vi "UT_002_TOML to LV.vi"() -> ()   [LabVIEW 2020]
uses:
  fb850d28-2e79-48d9-b60b-ba7296d5dbb4.vi
  89a8d650-8cb1-4c84-83d7-77e0f1707b6b.vi
  32d4b0e2-7f7c-42da-9dd6-c3c9d6f0c3e1.vi
  d279671c-9ecb-4521-8644-d889c2403450.vi
  5e8cb647-c85d-4476-b550-d09c056e5780.vi
  c4cfef05-1c91-402b-82a1-7a83dc25bed2.vi
  lib/TOML to LabVIEW.vi
  <vilib>/addons/_JKI Toolkits/Caraya/classes/Assert/Assert True.vi
  <vilib>/addons/_JKI Toolkits/Caraya/classes/Assert/Assert Not Error.vi
  <vilib>/addons/_JKI Toolkits/Caraya/classes/Assert/Assert Error.vi
  <vilib>/addons/_JKI Toolkits/Caraya/classes/Test/Test.lvclass
  <vilib>/addons/_JKI Toolkits/Caraya/classes/Assert/Assert.lvclass
  lib/TOML.lvlib
panel:
  out "error out":errorcluster
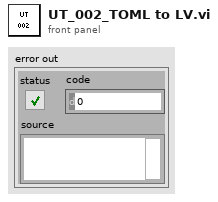
[diagram p1: front panel]
types:
  T1 = cluster{"cluster":cluster{"status":bool, "code":i32, "source":string, "error":errorcluster, "float-array":dbl[], "cluster-array":cluster{"nam":string, "value":dbl}[]}}
  T2 = cluster{"cluster":cluster{"status":bool, "cod":i32, "source":string, "error":errorcluster, "float-array":dbl[], "cluster-array":cluster{"name":string, "value":dbl}[]}}
  T3 = cluster{"status":bool, "code":i32, "source":string, "error":errorcluster, "float-array":dbl[], "cluster-array":cluster{"name":string, "value":dbl}[]}
  T4 = cluster{"cluster":cluster{"status":bool, "code":i32, "source":string, "error":errorcluster, "float-array":dbl[], "cluster-array":cluster{"name":string, "value":dbl}[]}}
  T5 = typedef "TOML.lvlib/TOML Value.ctl" = cluster{"type":enum16{"Table", "Array", "String", "Integer", "Float", "Boolean", "Offset Date-Time", "Local Date-Time", "Local Date", "Local Time", "Path"}, "value":variant}
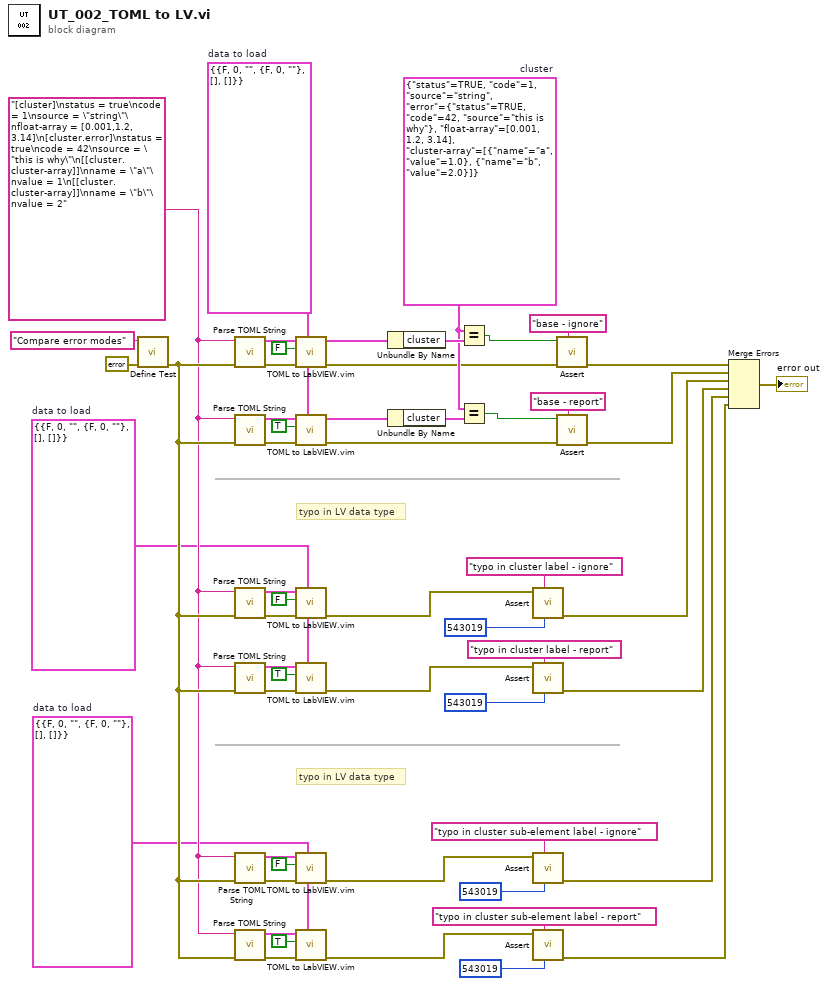
[diagram p0: block diagram]
diagram:
  w3 = T1 {"cluster"={"status"=FALSE, "code"=0, "source"="", "error"={"status"=FALSE, "code"=0, "source"=""}, "float-array"=[], "cluster-array"=[]}}  # data to load
  w10 = T2 {"cluster"={"status"=FALSE, "cod"=0, "source"="", "error"={"status"=FALSE, "code"=0, "source"=""}, "float-array"=[], "cluster-array"=[]}}  # data to load
  w30 = T3 {"status"=TRUE, "code"=1, "source"="string", "error"={"status"=TRUE, "code"=42, "source"="this is why"}, "float-array"=[0.001, 1.2, 3.14], "cluster-array"=[{"name"="a", "value"=1.0}, {"name"="b", "value"=2.0}]}  # cluster
  w26 = T4 {"cluster"={"status"=FALSE, "code"=0, "source"="", "error"={"status"=FALSE, "code"=0, "source"=""}, "float-array"=[], "cluster-array"=[]}}  # data to load
  w33 = "[cluster]\nstatus = true\ncode = 1\nsource = \"string\"\nfloat-array = [0.001,1.2, 3.14]\n[cluster.error]\nstatus = true\ncode = 42\nsource = \"this is why\"\n[[cluster.cluster-array]]\nname = \"a\"\nvalue = 1\n[[cluster.cluster-array]]\nname = \"b\"\nvalue = 2" ("String")
  # "typo in LV data type"
  # "typo in LV data type"
  n1 = call <vilib>:"Define Test.vi"("error in (no error)"=errorcluster {"status"=FALSE, "code"=0, "source"=""}, "Label (VI Title)"="Compare error modes") -> ("error out"=w34:errorcluster)  [unwired: 8 in, 1 out]
  n2 = call "Parse TOML String.vi"("error in (no error)"=w34, "String"=w33) -> ("error out"=w28:errorcluster, "Value"=w29:T5)  [unwired: 8 in]
  n3 = call "Parse TOML String.vi"("error in (no error)"=w34, "String"=w33) -> ("error out"=w27:errorcluster, "Value"=w25:T5)  [unwired: 8 in]
  n4 = call "Parse TOML String.vi"("error in (no error)"=w34, "String"=w33) -> ("error out"=w17:errorcluster, "Value"=w18:T5)  [unwired: 8 in]
  n5 = call "Parse TOML String.vi"("error in (no error)"=w34, "String"=w33) -> ("error out"=w13:errorcluster, "Value"=w14:T5)  [unwired: 8 in]
  n6 = call "Parse TOML String.vi"("error in (no error)"=w34, "String"=w33) -> ("error out"=w9:errorcluster, "Value"=w4:T5)  [unwired: 8 in]
  n7 = call "Parse TOML String.vi"("error in (no error)"=w34, "String"=w33) -> ("error out"=w7:errorcluster, "Value"=w5:T5)  [unwired: 8 in]
  n8 = call "TOML to LabVIEW.vim"("datatype"=w26, "error in (no error)"=w28, "Error if missing element"=FALSE, "Value"=w29) -> ("error out"=w21:errorcluster, "LV Data"=w22:T4)  [unwired: 5 in, 1 out]
  n9 = call "TOML to LabVIEW.vim"("datatype"=w26, "error in (no error)"=w27, "Error if missing element"=TRUE, "Value"=w25) -> ("error out"=w19:errorcluster, "LV Data"=w20:T4)  [unwired: 5 in, 1 out]
  n10 = call "TOML to LabVIEW.vim"("datatype"=w10, "error in (no error)"=w17, "Error if missing element"=FALSE, "Value"=w18) -> ("error out"=w15:errorcluster)  [unwired: 5 in, 2 out]
  n11 = call "TOML to LabVIEW.vim"("datatype"=w10, "error in (no error)"=w13, "Error if missing element"=TRUE, "Value"=w14) -> ("error out"=w11:errorcluster)  [unwired: 5 in, 2 out]
  n12 = call "TOML to LabVIEW.vim"("datatype"=w3, "error in (no error)"=w9, "Error if missing element"=FALSE, "Value"=w4) -> ("error out"=w8:errorcluster)  [unwired: 5 in, 2 out]
  n13 = call "TOML to LabVIEW.vim"("datatype"=w3, "error in (no error)"=w7, "Error if missing element"=TRUE, "Value"=w5) -> ("error out"=w6:errorcluster)  [unwired: 5 in, 2 out]
  n14 = Unbundle By Name(w22) -> ("cluster"=w49:T3)
  n15 = Unbundle By Name(w20) -> ("cluster"=w42:T3)
  n16 = Equal?(x=w30, y=w49) -> (x = y?=w51:bool)
  n17 = Equal?(x=w30, y=w42) -> (x = y?=w41:bool)
  n18 = call-poly <vilib>:"Assert.vi"("error code (1)"=543019, "Label"="typo in cluster label - ignore" ("Label (VI Title)"), "Not Error?"=w15) -> ("error out"=w47:errorcluster)  [unwired: 7 in, 1 out]
  n19 = call-poly <vilib>:"Assert.vi"("error code (1)"=543019, "Label"="typo in cluster label - report" ("Label (VI Title)"), "Error?"=w11) -> ("error out"=w31:errorcluster)  [unwired: 7 in, 1 out]
  n20 = call-poly <vilib>:"Assert.vi"("error code (1)"=543019, "Label"="typo in cluster sub-element label - ignore" ("Label (VI Title)"), "Not Error?"=w8) -> ("error out"=w45:errorcluster)  [unwired: 7 in, 1 out]
  n21 = call-poly <vilib>:"Assert.vi"("error code (1)"=543019, "Label"="typo in cluster sub-element label - report" ("Label (VI Title)"), "Error?"=w6) -> ("error out"=w32:errorcluster)  [unwired: 7 in, 1 out]
  n22 = call-poly <vilib>:"Assert.vi"("Label"="base - ignore" ("Label (VI Title)"), "error in (no error)"=w21, "True?"=w51) -> ("error out"=w54:errorcluster)  [unwired: 7 in, 1 out]
  n23 = call-poly <vilib>:"Assert.vi"("Label"="base - report" ("Label (VI Title)"), "error in (no error)"=w19, "True?"=w41) -> ("error out"=w39:errorcluster)  [unwired: 7 in, 1 out]
  n24 = Merge Errors(w54, w39, w47, w31, w45, w32) -> (→"error out":errorcluster)
